vi "Init.vi"(8 "error in (no error)":errorcluster, 10 "Instrument String":variant, 11 "KE65XX DMM in":refnum<class "Keithley 65XX DMM.lvclass">) -> (0 "error out":errorcluster, 2 "Found?":bool=TRUE, 3 "KE65XX DMM out":refnum<class "Keithley 65XX DMM.lvclass">)   [LabVIEW 2025, in "DMM.lvlib" / "Keithley 65XX DMM.lvclass"]
uses:
  Keithley 65XX DMM.lvclass
  C:/Working copy/tss/Plugin/Engines/DMM/DMM Instrument/DMM Instrument.lvclass
  DMM configuration/DMM configuration.lvclass
  C:/Users/Public/Documents/Sandia National Labs/TSS Plugin/Abstract Engine.lvlibp/Instrument configuration/Instrument configuration.lvclass
  Keithley 65XX DMM.lvclass/Keithley 65XX DMM.ctl
  Users/Public/Documents/Sandia National Labs/TSS Plugin/Abstract Engine.lvlibp/Instrument configuration/Read Instrument Setting.vi
  Users/Public/Documents/Sandia National Labs/TSS Plugin/CEF.lvlibp/serializable configuration/CEF_serializable configuration.lvclass
  <instrlib>/Keithley DMM6500 DAQ6500 Series/Keithley DMM6500 DAQ6500 Series.lvlib
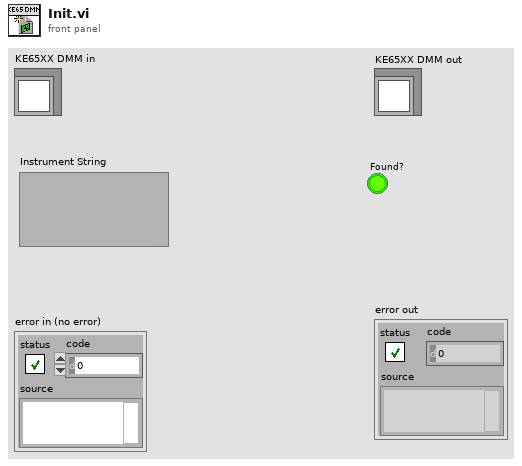
[diagram p1: front panel]
types:
  T1 = typedef "Abstract Engine.lvlibp/Instrument configuration.lvclass/Default Instrument.ctl" = cluster{"Type":string, "Address":string, "SW Alias":string, "Description":string, "Enabled":bool}
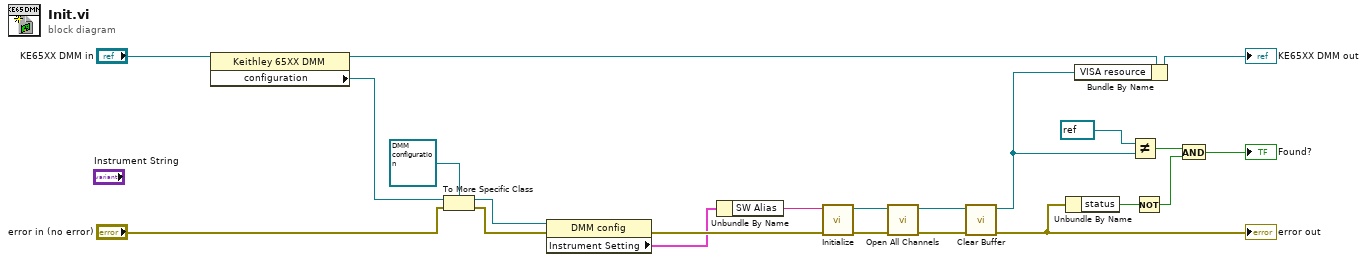
[diagram p0: block diagram]
diagram:
  n1 = property class="Keithley 65XX DMM"(reference="KE65XX DMM in") -> (reference out=w16:refnum<class "Keithley 65XX DMM.lvclass">, "configuration"=w11:refnum<class "CEF_serializable configuration.lvclass">)  [unwired: 1 in, 1 out]
  n2 = To More Specific Class(target class=refnum<class "DMM configuration.lvclass"> refnum ("DMM.lvlib:DMM configuration.lvclass"), reference=w11, error in="error in (no error)") -> (specific class reference=w12:refnum<class "DMM configuration.lvclass">, error out=w13:errorcluster)
  n3 = property class="DMM config"(reference=w12, error in=w13) -> (error out=w8:errorcluster, "Instrument Setting"=w1:T1)  [unwired: 1 out]
  n4 = Unbundle By Name(w1) -> ("SW Alias"=w10:string)
  n5 = call <instrlib>:"Initialize.vi"("error in (no error)"=w8, "VISA resource name"=w10) -> ("error out"=w21:errorcluster, "VISA resource name out"=w20:refnum<visa-resource-name>)  [unwired: 8 in]
  n6 = call <instrlib>:"Open All Channels.vi"("error in (no error)"=w21, "VISA resource name"=w20) -> ("error out"=w19:errorcluster, "VISA resource name out"=w18:refnum<visa-resource-name>)  [unwired: 8 in]
  n7 = call <instrlib>:"Clear Buffer.vi"("error in (no error)"=w19, "VISA resource name"=w18) -> ("error out"=w5:errorcluster, "VISA resource name out"=w14:refnum<visa-resource-name>)  [unwired: 8 in]
  "error out" <- w5
  n8 = Unbundle By Name(w5) -> ("status"=w6:bool)
  n9 = Bundle By Name(cluster=w16, "VISA resource"=w14) -> (→"KE65XX DMM out":refnum<class "Keithley 65XX DMM.lvclass">)
  n10 = Not Equal?(x=refnum<visa-resource-name> refnum ("VISA resource name out"), y=w14) -> (x != y?=w4:bool)
  n11 = Not(x=w6) -> (.not. x?=w3:bool)
  n12 = And(x=w4, y=w3) -> (x .and. y?=→"Found?":bool)
